vi "Untitled 3.vi"(7 "Boolean":bool, 10 "concatenated":string, 11 "Direct program":T1) -> (2 "value":T1, 3 "concatenated string":string)   [LabVIEW 2015]
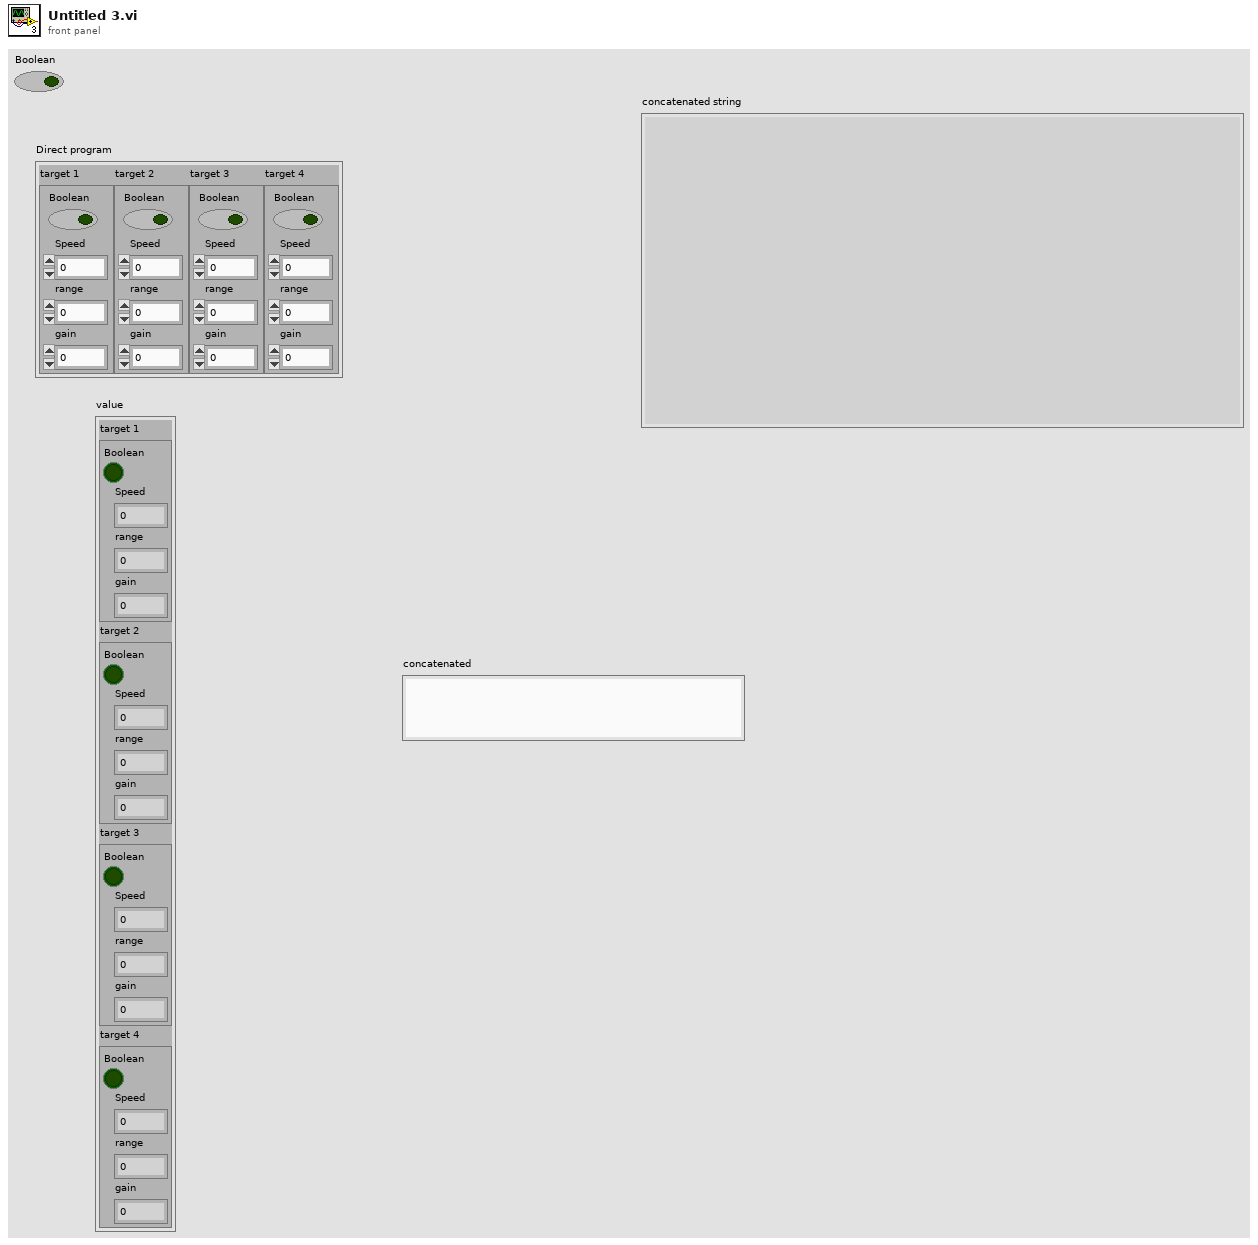
[diagram p1: front panel]
types:
  T1 = cluster{"target 1":cluster{"Boolean":bool, "Speed":dbl, "range":dbl, "gain":dbl}, "target 2":cluster{"Boolean":bool, "Speed":dbl, "range":dbl, "gain":dbl}, "target 3":cluster{"Boolean":bool, "Speed":dbl, "range":dbl, "gain":dbl}, "target 4":cluster{"Boolean":bool, "Speed":dbl, "range":dbl, "gain":dbl}}
  T2 = cluster{"Boolean":bool, "Speed":dbl, "range":dbl, "gain":dbl}[]
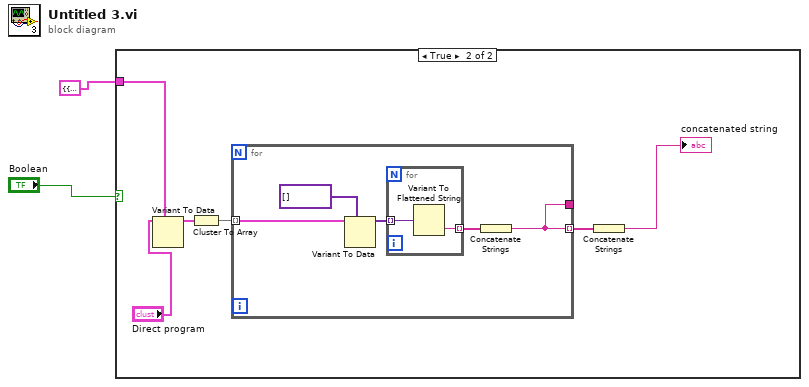
[diagram p0: block diagram]
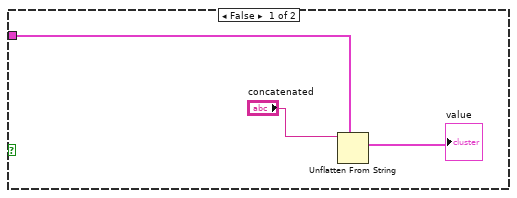
[diagram p2: hidden frame]
diagram:
  n1 = case shown="True" "Boolean" {
    tunnel: T1 {"target 1"={"Boolean"=FALSE, "Speed"=0.0, "range"=0.0, "gain"=0.0}, "target 2"={"Boolean"=FALSE, "Speed"=0.0, "range"=0.0, "gain"=0.0}, "target 3"={"Boolean"=FALSE, "Speed"=0.0, "range"=0.0, "gain"=0.0}, "target 4"={"Boolean"=FALSE, "Speed"=0.0, "range"=0.0, "gain"=0.0}} ("Direct program 2") -> [w4 w7]
    frame False {
      n2 = Unflatten From String(type=w4, binary string="concatenated") -> (value=→"value":T1)  [unwired: 3 in, 2 out]
    }
    frame True {
      n3 = Variant To Data(type=w7, Variant="Direct program") -> (data=w11:T1)  [unwired: 1 in, 1 out]
      n4 = Cluster To Array(cluster=w11) -> (array=w10:T2)
      n5 = for {
        tunnel: w10 -> [w14] mode=indexing
        tunnel: [w12] -> w9 mode=indexing
        tunnel: [w12] -> _
        n6 = Variant To Data(type=variant[] [], Variant=w14) -> (data=w15:variant[])  [unwired: 1 in, 1 out]
        n7 = for {
          tunnel: w15 -> [w18] mode=indexing
          tunnel: [w17] -> w13 mode=indexing
          n8 = Variant To Flattened String(Variant=w18) -> (data string=w17:string)  [unwired: 1 out]
        }
        n9 = Concatenate Strings(w13) -> (w12:string)
      }
      n10 = Concatenate Strings(w9) -> (→"concatenated string":string)
    }
  }
